vi "2022_day06_sub_serach.vi"(9 "# of consecutive unique characters":i32, 11 "Puzzle Input Data":string) -> (1 "Msg Position":i32, 2 "Found?":bool)   [LabVIEW 2021]
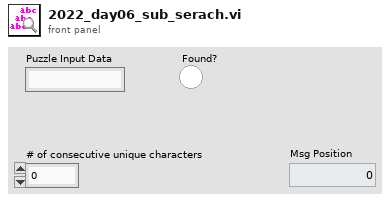
[diagram p1: front panel]
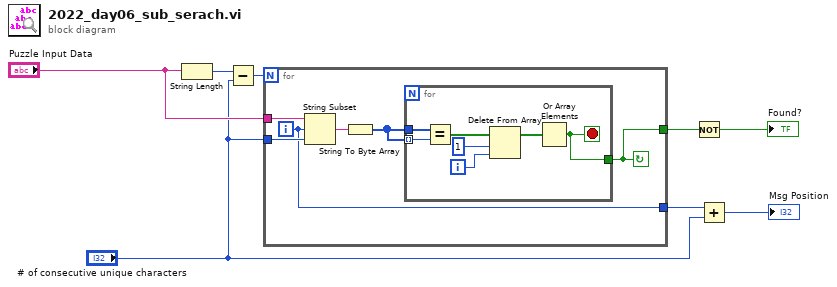
[diagram p0: block diagram]
diagram:
  n1 = String Length(string="Puzzle Input Data") -> (length=w1:i32)
  n2 = Subtract(x=w1, y="# of consecutive unique characters") -> (x-y=w2:i32)
  n3 = for {
    N: w2 -> [_]
    tunnel: "Puzzle Input Data" -> [w14]
    tunnel: "# of consecutive unique characters" -> [w13]
    tunnel: [w10] -> w3
    tunnel: [w9] -> w7
    i -> [w10]
    stop <- w9 continue-if-true
    n4 = String Subset(string=w14, offset (0)=w10, length (rest)=w13) -> (substring=w12:string)
    n5 = String To Byte Array(string=w12) -> (unsigned byte array=w11:u8[])
    n6 = for {
      tunnel: w11 -> [w20]
      tunnel: w11 -> [w21] mode=indexing
      tunnel: [w18] -> w9
      i -> [w16]
      stop <- w18 stop-if-true
      n7 = Equal?(x=w20, y=w21) -> (x = y?=w19:bool[])
      n8 = Delete From Array(array=w19, length=1, index=w16) -> (array with subset deleted=w17:bool[])  [unwired: 1 out]
      n9 = Or Array Elements(Boolean array=w17) -> (logical OR=w18:bool)
    }
  }
  n10 = Not(x=w7) -> (.not. x?=→"Found?":bool)
  n11 = Add(x=w3, y="# of consecutive unique characters") -> (x+y=→"Msg Position":i32)
